vi "Status Reporting.vi"(0 "VISA resource name":refnum<visa-resource-name>, 9 "?":bool, 11 "error in (no error)":errorcluster) -> (3 "event status register":bool[](array[boolean]), 4 "VISA resource name out":refnum<visa-resource-name>, 8 "status byte":bool[](array[boolean]), 10 "event status register B":bool[](array[boolean]), 15 "error out":errorcluster)   [LabVIEW 2018, in "Agilent 87XX Series.lvlib"]
doc: "This VI for the HP8753B Network Analyzer reads the status byte and the two event status registers. The two status registers are read out as regular output and will therefore clear anything already in the output queue."
uses:
  Agilent 87XX Series.lvlib
panel:
  # "read status byte only\nread status byte and status registers"
  # "Single, Num of Groups, or Cal Standard Complete\n\nService Routine Waiting\n\nData Entry Complete\n\nLimit Failed CH 2\n\nLimit Failed CH 1\n\nSearch Fail CH 2\n\nSearch Fail CH 1\n\nALC Unlock"
  # "Operation Complete\n\nRequest Control\n\nQuery Error\n\n\n\nExecution Error\n\nSyntax Error (GP-IB)\n\nUser Request\n\nPower On"
  # "Reverse GET\n\nForward GET\n\nEvent Status Register B\n\nCheck Error Queue\n\nMessage in Output Queue\n\nEvent Status Register\n\nRequest Service"
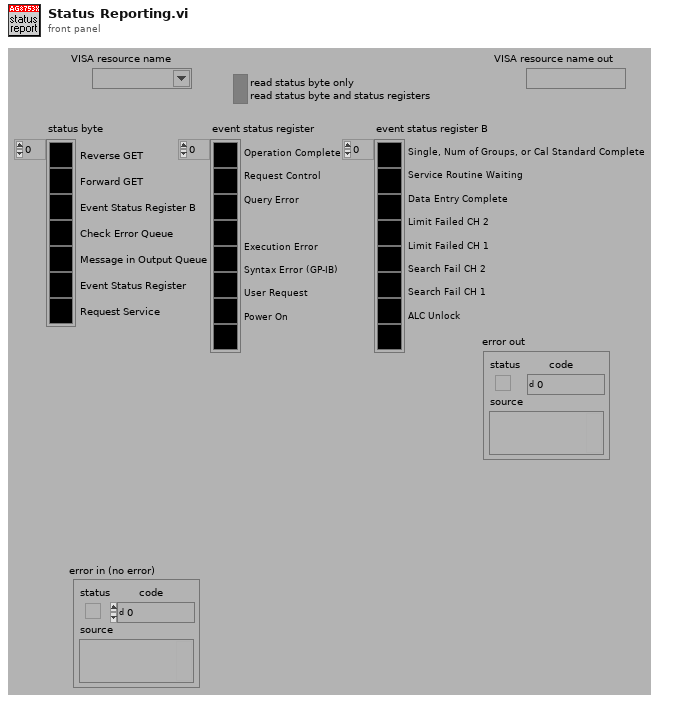
[diagram p1: front panel]
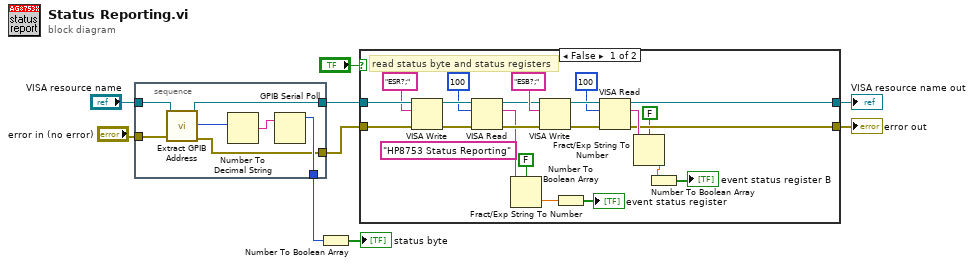
[diagram p0: block diagram]
diagram:
  n1 = stacked-sequence {
    tunnel: [w15] -> w8
    tunnel: "VISA resource name" -> [w13]
    tunnel: [w12] -> w5
    tunnel: [w11] -> w2
    tunnel: "error in (no error)" -> [w10]
    frame #0 {
      n2 = call "Extract GPIB Address.VI"("error in (no error)"=w10, "VISA resource name"=w13) -> ("error out"=w11:errorcluster, "GPIB address"=w14:u16, "VISA resource name out"=w12:refnum<visa-resource-name>)  [unwired: 6 in, 1 out]
      n3 = Number To Decimal String(number=w14) -> (decimal integer string=w16:string)  [unwired: 1 in]
      n4 = GPIB Serial Poll(0:w16) -> (2:w15:i16)  [unwired: 1 in, 2 out]
    }
  }
  n5 = Number To Boolean Array(number=w8) -> (Boolean array=→"status byte":bool[])
  n6 = case shown="False" "?" {
    tunnel: w5 -> [w37 w40]
    tunnel: w2 -> [w38 w39]
    tunnel: [w24 w40] -> w4
    tunnel: [w23 w39] -> w3
    frame False {
      (unwired) "HP8753 Status Reporting"
      # "read status byte and status registers"
      n7 = VISA Write(VISA resource name=w37, write buffer="ESR?;", error in (no error)=w38) -> (VISA resource name out=w20:refnum<visa-resource-name>, error out=w27:errorcluster)  [unwired: 1 out]
      n8 = VISA Read(VISA resource name=w20, byte count=100, error in (no error)=w27) -> (VISA resource name out=w32:refnum<visa-resource-name>, read buffer=w25:string, error out=w33:errorcluster)  [unwired: 1 out]
      n9 = Fract/Exp String To Number(use system decimal point (T)=FALSE, string=w25) -> (number=w26:dbl)  [unwired: 2 in, 1 out]
      n10 = VISA Write(VISA resource name=w32, write buffer="ESB?;", error in (no error)=w33) -> (VISA resource name out=w22:refnum<visa-resource-name>, error out=w29:errorcluster)  [unwired: 1 out]
      n11 = Number To Boolean Array(number=w26) -> (Boolean array=→"event status register":bool[])
      n12 = VISA Read(VISA resource name=w22, byte count=100, error in (no error)=w29) -> (VISA resource name out=w24:refnum<visa-resource-name>, read buffer=w31:string, error out=w23:errorcluster)  [unwired: 1 out]
      n13 = Fract/Exp String To Number(use system decimal point (T)=FALSE, string=w31) -> (number=w30:dbl)  [unwired: 2 in, 1 out]
      n14 = Number To Boolean Array(number=w30) -> (Boolean array=→"event status register B":bool[])
    }
    frame True {
      # "read status byte only"
    }
  }
  "VISA resource name out" <- w4
  "error out" <- w3
